vi "DAC Array to String.vi"(1 "6713 Write":dbl[](array[numeric])=[5.0, 9.199999809265137, 1.0, 6.699999809265137, 41.0, 42.0, -4.0, -8.0] format="%.2f") -> (0 "string":string)   [LabVIEW 2013]
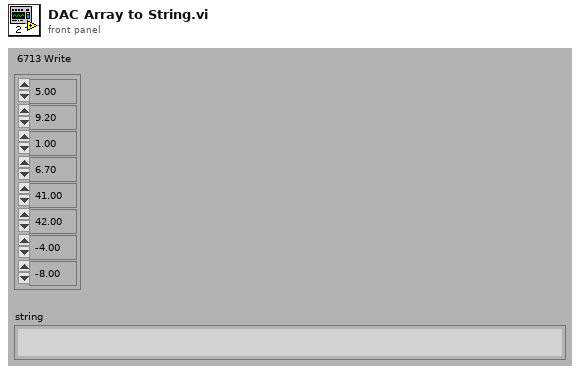
[diagram p1: front panel]
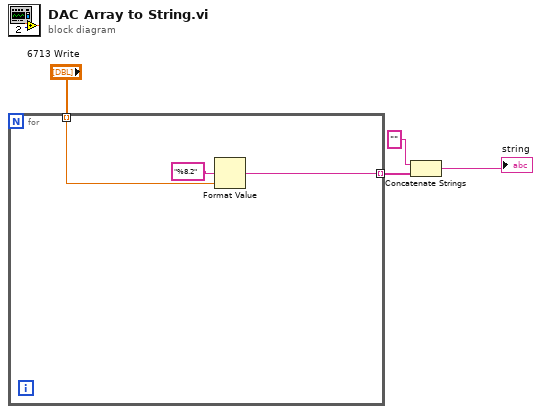
[diagram p0: block diagram]
diagram:
  n1 = for {
    tunnel: "6713 Write" -> [w6] mode=indexing
    tunnel: [w5] -> w2 mode=indexing
    n2 = Format Value(format string="%8.2", value (0)=w6) -> (output string=w5:string)  [unwired: 1 in]
  }
  n3 = Concatenate Strings("" ("string"), w2) -> (→"string":string)
